vi "Activity Light - TEST.vi"() -> ()   [LabVIEW 2024, in "EQMF.lvlib" / "Status Utils.lvlib"]
uses:
  Status Utils.lvlib
  Activity Light Color Types.ctl
panel:
  in  "Duration(ms)":u32=100
  in  "Set Pulse Dur":bool
  in  "OFF Color":u32(colorbox)=16722656
  in  "ON Color":u32(colorbox)=16722656
  in  "Type":T1=enum."Active (Yellow)"
  out "Progress":i32(slide) scale=0.0..50.0
  in  "Pulse 50":bool
  out "Active":bool
  in  "Exit":bool
  in  "Pulse":bool
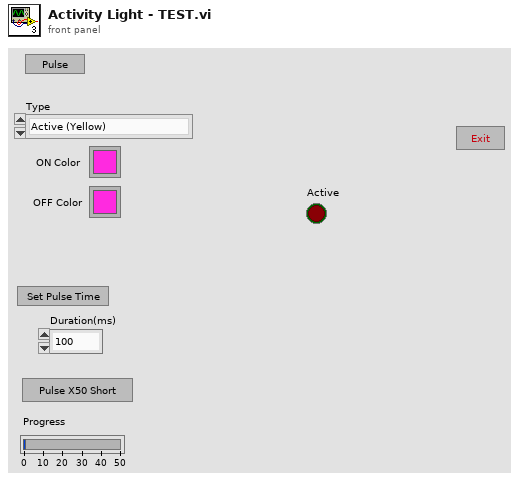
[diagram p1: front panel]
types:
  T1 = typedef "EQMF.lvlib/Status Utils.lvlib/Activity Light Color Types.ctl" = enum16{"OK (Green)", "Active (Yellow)", "Warning (Orange)", "Error (Red)", "Attention (Blue)", "Custom Color"}
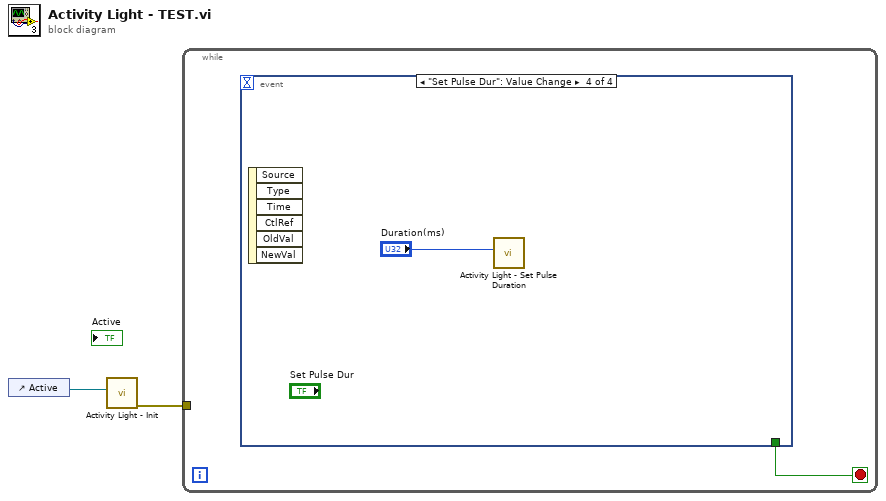
[diagram p0: block diagram]
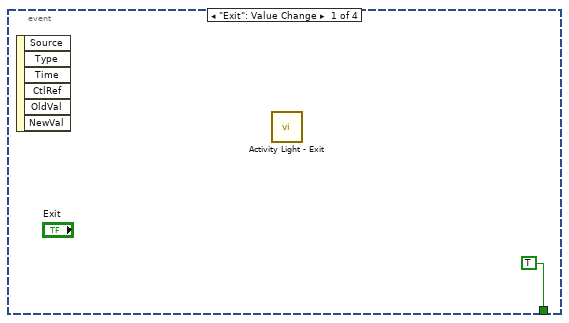
[diagram p2: hidden frame]
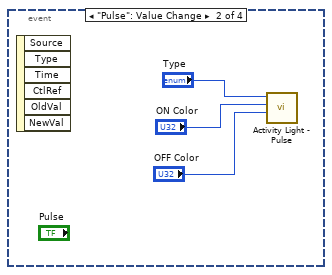
[diagram p3: hidden frame]
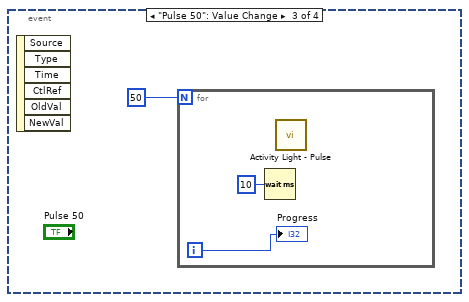
[diagram p4: hidden frame]
diagram:
  n1 = control-ref of="Active"() -> (w2:refnum<vi>)
  n2 = call "Activity Light - Init.vi"("Boolean LED"=w2) -> ("error out"=w1:errorcluster)  [unwired: 9 in, 1 out]
  n3 = while {
    tunnel: w1 -> [_]
    stop <- w3 stop-if-true
    n4 = event shown="[3] \"Set Pulse Dur\": Value Change" {
      selector: _ -> [_ _ _ _]
      dyn-events: _ -> [_ _ _ _]
      timeout: _ -> [_ _ _ _]
      tunnel: [TRUE _ _ _] -> w3
      event "Exit": Value Change {
        n5 = event-data() -> ()  [unwired: 1 in, 6 out]
        n6 = call "Activity Light - Exit.vi"() -> ()  [unwired: 11 in, 1 out]
      }
      event "Pulse": Value Change {
        n7 = event-data() -> ()  [unwired: 1 in, 6 out]
        n8 = call "Activity Light - Pulse.vi"("OFF Color"="OFF Color", "ON Color"="ON Color", "Type"="Type") -> ()  [unwired: 8 in, 1 out]
      }
      event "Pulse 50": Value Change {
        n9 = event-data() -> ()  [unwired: 1 in, 6 out]
        n10 = for {
          N: 50 -> [_]
          i -> [w9]
          n11 = Wait (ms)(milliseconds to wait=u32 10) -> ()  [unwired: 1 out]
          n12 = call "Activity Light - Pulse.vi"() -> ()  [unwired: 11 in, 1 out]
          "Progress" <- w9
        }
      }
      event "Set Pulse Dur": Value Change {
        n13 = event-data() -> ()  [unwired: 1 in, 6 out]
        n14 = call "Activity Light - Set Pulse Duration.vi"("Duration(ms)"="Duration(ms)") -> ()  [unwired: 10 in, 1 out]
      }
    }
  }
